vi "Start Streaming.vi"(8 "error in (no error)":errorcluster, 9 "Camera Settings":T1={"Exposure Time (ms)"=100.0, "Binning"=enum."2x2", "Scan Mode"=-1, "Frames to Acquire"=1000.0, "Pixel Correction"=FALSE, "Frames to Skip"=1, "File Path"=path "", "Duty cycle"=1.0, "ALEX"=FALSE, "Shutter Enable"=[], "fluidics trigger frame"=0, "Bit Depth"=16, "Image Width (px)"=0, "Image Height (px)"=0, "Horizontal Offset (px)"=0, "Vertical Offset (px)"=0} {"fluidics trigger frame" max=60000 step=1; "Exposure Time (ms)" min=1.0 max=10000.0 step=1.0}, 11 "Synchronization Device in":refnum<class "NI DAQ.lvclass">) -> (0 "error out":errorcluster, 3 "Synchronization Device out":refnum<class "NI DAQ.lvclass">)   [LabVIEW 2023, in "NI DAQ.lvlib" / "NI DAQ.lvclass"]
uses:
  NI DAQ.lvclass
  Resources/Type Defs/Camera Settings.ctl
  NI DAQ.lvclass/NI DAQ.ctl
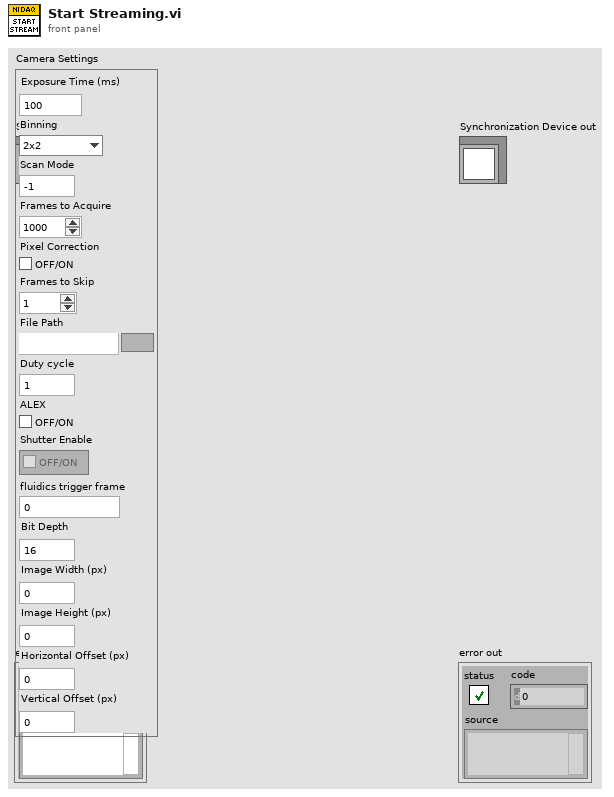
[diagram p1: front panel]
types:
  T1 = typedef "Camera Settings.ctl" = cluster{"Exposure Time (ms)":dbl, "Binning":enum16{"1x1", "2x2", "4x4"}, "Scan Mode":i32, "Frames to Acquire":dbl, "Pixel Correction":bool, "Frames to Skip":u32, "File Path":path, "Duty cycle":dbl, "ALEX":bool, "Shutter Enable":bool[], "fluidics trigger frame":u16, "Bit Depth":u16, "Image Width (px)":u16, "Image Height (px)":u16, "Horizontal Offset (px)":u16, "Vertical Offset (px)":u16}
  T2 = typedef "sync device settings.ctl" = cluster{"Interval (ms)":dbl, "ALEX":bool, "Shutter Enable":bool[], "Stream":bool, "Duty Cycle":dbl, "fluidics trigger frame":u16, "Frames to Skip":u32}
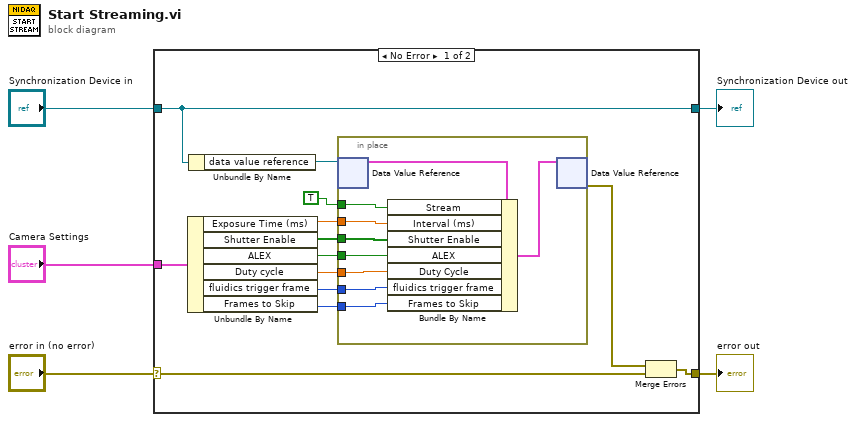
[diagram p0: block diagram]
diagram:
  n1 = case shown="No Error" "error in (no error)" {
    selector: "error in (no error)" -> [w16 w29]
    tunnel: [w17 w29] -> w4
    tunnel: [w18 w28] -> w2
    tunnel: "Synchronization Device in" -> [w18 w28]
    tunnel: "Camera Settings" -> [w13 _]
    frame No Error {
      n2 = Unbundle By Name(w13) -> ("Exposure Time (ms)"=w12:dbl, "Shutter Enable"=w11:bool[], "ALEX"=w10:bool, "Duty cycle"=w9:dbl, "fluidics trigger frame"=w8:u16, "Frames to Skip"=w7:u32)
      n3 = Unbundle By Name(w18) -> ("data value reference"=w15:refnum<data-value>)
      n4 = in-place {
        in-place-border: TRUE ("Streaming?") -> [w26]
        in-place-border: w12 -> [w24]
        in-place-border: w9 -> [w23]
        in-place-border: w10 -> [w22]
        in-place-border: w11 -> [w21]
        in-place-border: w8 -> [w20]
        in-place-border: w7 -> [w19]
        n5 = in-place-dvr #1(w15) -> (w25:T2)  [unwired: 1 out]
        n6 = Bundle By Name(cluster=w25, "Stream"=w26, "Interval (ms)"=w24, "Shutter Enable"=w21, "ALEX"=w22, "Duty Cycle"=w23, "fluidics trigger frame"=w20, "Frames to Skip"=w19) -> (w27:T2)
        n7 = in-place-dvr #1(w27) -> (w14:errorcluster)  [unwired: 1 out]
      }
      n8 = Merge Errors(w14, w16) -> (w17:errorcluster)
    }
    frame Error {
    }
  }
  "error out" <- w4
  "Synchronization Device out" <- w2
